vi "sublijncode.vi"() -> (1 "Boolean":bool, 2 "Array 2":i32[](array[numeric]), 3 "appended array":dbl[](array[numeric]), 4 "Array":i32[](array[numeric]))   [LabVIEW 2019]
uses:
  <vilib>/myRIO/Common/Instrument Driver Framework/Utilities/typedefs/Analog Scaling Constants.ctl
  <vilib>/myRIO/Common/Instrument Driver Framework/Utilities/typedefs/Analog Scaling Constants List.ctl
  <vilib>/myRIO/Common/Instrument Driver Framework/myRIO v1.0/AI/typedefs/AI Channels Enum.ctl
  <vilib>/myRIO/Common/Instrument Driver Framework/myRIO v1.0/AI/typedefs/AI Channels List.ctl
  <vilib>/myRIO/Common/Instrument Driver Framework/Utilities/typedefs/Generic FPGA Reference.ctl
  <vilib>/myRIO/Common/Instrument Driver Framework/Utilities/typedefs/myRIO v1.0 Reference.ctl
  <vilib>/myRIO/Common/Instrument Driver Framework/Utilities/typedefs/Hardware Version Enum.ctl
  <vilib>/myRIO/Common/Instrument Driver Framework/Utilities/typedefs/myRIO Generic Hardware Reference.ctl
  <vilib>/myRIO/Instrument Drivers/Onboard IO/AI/typedefs/AI Reference.ctl
  <vilib>/myRIO/Instrument Drivers/Onboard IO/AI/AI.lvlib
  <vilib>/myRIO/Instrument Drivers/Onboard IO/AI/vis/Read.vi
  <vilib>/userDefined/High Color/nirio_resource_hc.ctl
  <vilib>/myRIO/Common/Instrument Driver Framework/myRIO v1.0/AI/vis/myRIO v1.1 Open AI.vi
  <vilib>/myRIO/Instrument Drivers/Onboard IO/AI/vis/myRIO AI Open.xnode
  <vilib>/myRIO/Common/Instrument Driver Framework/Utilities/vis/Is FPGA Ref Available.vi
  <vilib>/myRIO/Express VI/Onboard IO/AI/AI Express VI.xnode
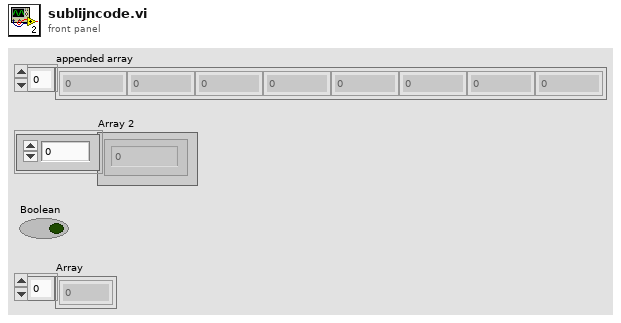
[diagram p1: front panel]
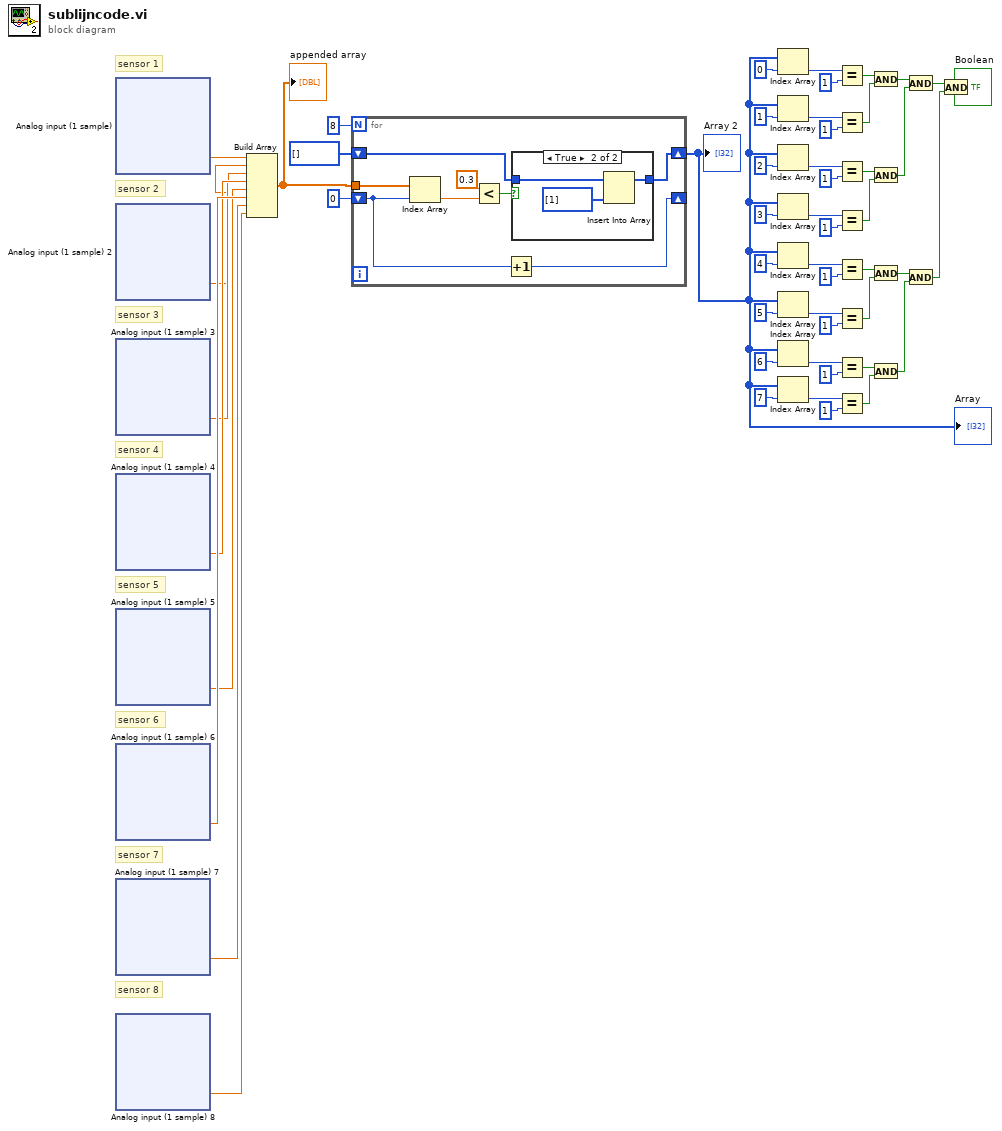
[diagram p0: block diagram]
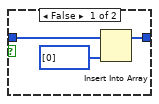
[diagram p2: hidden frame]
diagram:
  # "sensor 8"
  # "sensor 7"
  # "sensor 6"
  # "sensor 5"
  # "sensor 4"
  # "sensor 3"
  # "sensor 2"
  # "sensor 1"
  n1 = xnode "Analog input (1 sample)"() -> ("A/AI3 (Pin 9)"=w44:dbl)  [unwired: 1 in, 1 out]
  n2 = xnode "Analog input (1 sample) 2"() -> ("A/AI2 (Pin 7)"=w45:dbl)  [unwired: 1 in, 1 out]
  n3 = xnode "Analog input (1 sample) 3"() -> ("A/AI1 (Pin 5)"=w46:dbl)  [unwired: 1 in, 1 out]
  n4 = xnode "Analog input (1 sample) 4"() -> ("A/AI0 (Pin 3)"=w47:dbl)  [unwired: 1 in, 1 out]
  n5 = xnode "Analog input (1 sample) 5"() -> ("B/AI3 (Pin 9)"=w48:dbl)  [unwired: 1 in, 1 out]
  n6 = xnode "Analog input (1 sample) 6"() -> ("B/AI2 (Pin 7)"=w49:dbl)  [unwired: 1 in, 1 out]
  n7 = xnode "Analog input (1 sample) 7"() -> ("A/AI1 (Pin 5)"=w50:dbl)  [unwired: 1 in, 1 out]
  n8 = xnode "Analog input (1 sample) 8"() -> ("B/AI0 (Pin 3)"=w51:dbl)  [unwired: 1 in, 1 out]
  n9 = Build Array(w44, w45, w46, w47, w48, w49, w50, w51) -> (w52:dbl[])
  "appended array" <- w52
  n10 = for {
    N: 8 -> [_]
    shift-right: [w59] -> w1
    shift-left: i32[] [] -> [w60]
    shift-right: [w57] -> _
    shift-left: 0 -> [w54]
    tunnel: w52 -> [w55]
    n11 = Index Array(array=w55, index=w54) -> (element=w56:dbl)
    n12 = Less?(x=0.3, y=w56) -> (x < y?=w58:bool)
    n13 = Increment(x=w54) -> (x+1=w57:i32)
    n14 = case shown="True" w58 {
      tunnel: w60 -> [w62 w64]
      tunnel: [w63 w66] -> w59
      frame False {
        n15 = Insert Into Array(array=w62, new element=i32[] [0]) -> (w63:i32[])  [unwired: 1 in]
      }
      frame True {
        n16 = Insert Into Array(array=w64, new element=i32[] [1]) -> (w66:i32[])  [unwired: 1 in]
      }
    }
  }
  "Array 2" <- w1
  "Array" <- w1
  n17 = Index Array(array=w1, index=0) -> (element=w22:i32)
  n18 = Index Array(array=w1, index=1) -> (element=w43:i32)
  n19 = Index Array(array=w1, index=2) -> (element=w37:i32)
  n20 = Index Array(array=w1, index=3) -> (element=w40:i32)
  n21 = Index Array(array=w1, index=4) -> (element=w34:i32)
  n22 = Index Array(array=w1, index=5) -> (element=w31:i32)
  n23 = Index Array(array=w1, index=6) -> (element=w28:i32)
  n24 = Index Array(array=w1, index=7) -> (element=w25:i32)
  n25 = Equal?(x=w22, y=1) -> (x = y?=w19:bool)
  n26 = Equal?(x=w43, y=1) -> (x = y?=w18:bool)
  n27 = Equal?(x=w37, y=1) -> (x = y?=w17:bool)
  n28 = Equal?(x=w40, y=1) -> (x = y?=w16:bool)
  n29 = Equal?(x=w34, y=1) -> (x = y?=w15:bool)
  n30 = Equal?(x=w31, y=1) -> (x = y?=w14:bool)
  n31 = Equal?(x=w28, y=1) -> (x = y?=w13:bool)
  n32 = Equal?(x=w25, y=1) -> (x = y?=w12:bool)
  n33 = And(x=w19, y=w18) -> (x .and. y?=w11:bool)
  n34 = And(x=w17, y=w16) -> (x .and. y?=w10:bool)
  n35 = And(x=w15, y=w14) -> (x .and. y?=w9:bool)
  n36 = And(x=w13, y=w12) -> (x .and. y?=w8:bool)
  n37 = And(x=w11, y=w10) -> (x .and. y?=w7:bool)
  n38 = And(x=w9, y=w8) -> (x .and. y?=w6:bool)
  n39 = And(x=w7, y=w6) -> (x .and. y?=→"Boolean":bool)
